vi "XIPIN_AXI_BRAM_Controller_4_0.vi"   [LabVIEW 2017]
doc: "The AXI Block RAM (BRAM) Controller is a soft IP core. The core is designed as an AXI Endpoint slave IP for integration with the AXI interconnect and system master devices to communicate to local block RAM. The core supports both single and burst transactions to the block RAM and is optimized for performance.\n------------------------------------\n<b>Need License</b> : No\n<b>Interface</b> : AXI4"
uses:
  <vilib>/rvi/XilinxIP/XIPIN_XNode/niFpgaXIPIN.xnode
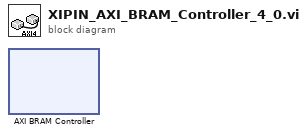
[diagram p0: block diagram]
diagram:
  n1 = xnode ("AXI BRAM Controller")() -> ()
